vi "QPosition.vi"(8 "error in (no error)":errorcluster, 10 "Axis":i32=1, 11 "VISA resource name in":refnum<visa-resource-name>) -> (0 "error out":errorcluster, 2 "Position":dbl, 3 "VISA resource name out":refnum<visa-resource-name>)   [LabVIEW 2019]
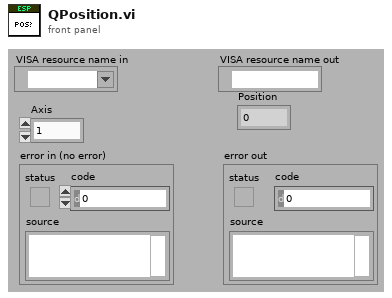
[diagram p1: front panel]
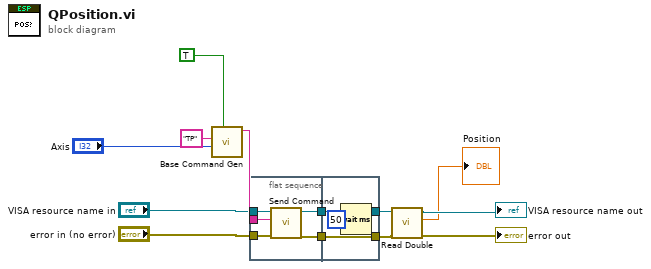
[diagram p0: block diagram]
diagram:
  n1 = call "Base Command Gen.vi"("Query"=TRUE, "Command"="TP", "xx"="Axis") -> ("Command"=w12:string)  [unwired: 8 in]
  n2 = flat-sequence {
    tunnel: "error in (no error)" -> [w18]
    tunnel: w12 -> [w17]
    tunnel: "VISA resource name in" -> [w16]
    tunnel: [w15] -> w3
    tunnel: [w14] -> w2
    tunnel: [w20] -> w6
    tunnel: [w21] -> w7
    tunnel: w3 -> [w21]
    tunnel: w2 -> [w20]
    frame #0 {
      n3 = call "Send Command.vi"("error out (no error)"=w18, "Command"=w17, "VISA resource name in"=w16) -> ("error out"=w14:errorcluster, "VISA resource name out"=w15:refnum<visa-resource-name>)  [unwired: 7 in]
    }
    frame #1 {
      n4 = Wait (ms)(milliseconds to wait=u32 50) -> ()  [unwired: 1 out]
    }
  }
  n5 = call "Read Double.vi"("error in (no error)"=w6, "VISA resource name"=w7) -> ("error out"=→"error out":errorcluster, "Double"=→"Position":dbl, "VISA resource name out"=→"VISA resource name out":refnum<visa-resource-name>)  [unwired: 7 in]
